vi "get_attrs.vi"() -> ()   [LabVIEW 2014]
uses:
  lvnanomsg/nanomsg.lvlib
panel:
  out "size":i32
  out "Array":i32[](array[numeric])
  in  "Cluster":T1
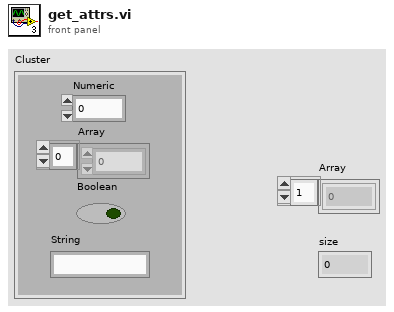
[diagram p1: front panel]
types:
  T1 = cluster{"Numeric":dbl, "Array":dbl[], "Boolean":bool, "String":string}
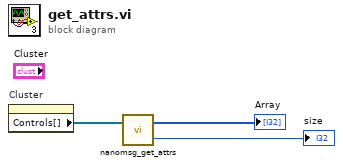
[diagram p0: block diagram]
diagram:
  n1 = property on="Cluster" class="Clust (strict)"() -> ("Controls[]"=w3:refnum<vi>[])  [unwired: 2 in, 2 out]
  n2 = call "nanomsg_get_attrs.vi"("ref array"=w3) -> ("size"=→"size":i32, "attrs"=→"Array":i32[])  [unwired: 1 in]
